vi "Wait For (str) (SubVI).vi"(1 "簇":T1={"initialize"=enum."SR830", "6221"={"6221 Resource"="GPIB0::24::INSTR", "Delta status"=FALSE, "电流"=0.0}, "SR830+6221"={"source"=0, "阻抗"=0.0, "量程入 4"=0, "量程入 3"=0, "量程入 2"=0, "量程入 1"=0, "SR830 2"=FALSE, "SR830 3"=FALSE, "SR830 4"=FALSE, "SR830 1"=FALSE, "VISA 1"="", "VISA 2"="", "VISA 3"="", "VISA 4"="", "Reserve 1"=0, "Reserve 2"=-1, "Reserve 3"=-1, "Reserve 4"=-1, "量程"=enum."量程每次测量会判定"}, "2400"={"2400"=FALSE, "VISA"=""}, "ch"={"ch"=[], "current"=[], "change?"=[], "holding current\nwhen change ch?"=FALSE}, "Instrument"={"335 Resource"="GPIB0::24::INSTR", "Input (0:A)"=0, "Instrument Type"=enum."SVSM", "quantum design"=refnum, "Heater Output (1:1)"=1, "semaphore"=refnum, "TCP master instance"=refnum, "335 Status"=refnum, "M24C Resource"="GPIB0::24::INSTR", "4G supply"="GPIB0::24::INSTR", "Temp Status 24C"=refnum, "4g supply status"=refnum, "Temp"=refnum}, "Aborting"=refnum, "数据文件"=refnum} {"Instrument"."Input (0:A)" items=["A", "B"]; "Instrument"."Heater Output (1:1)" items=["1"=1, "2"=2]; "SR830+6221"."Reserve 4" items=["Auto Reserve"=-1, "High Reserve"=0, "Normal"=1, "Low Noise"=2]; "SR830+6221"."Reserve 3" items=["Auto Reserve"=-1, "High Reserve"=0, "Normal"=1, "Low Noise"=2]; "SR830+6221"."Reserve 2" items=["Auto Reserve"=-1, "High Reserve"=0, "Normal"=1, "Low Noise"=2]; "SR830+6221"."Reserve 1" items=["量程每次测量会判定", "量程不变为设定值"]; "SR830+6221"."source" items=["SR830 1", "SR830 2", "SR830 3", "SR830 4"]}, 2 "字符串":string, 3 "error out":errorcluster) -> (10 "错误输出":errorcluster)   [LabVIEW 2019, in "Take Seq.lvlib"]
uses:
  Take Seq.lvlib
  <vilib>/NI/Modbus Library/API/Master/Modbus Master.lvclass
  config.ctl
  initialize.ctl
  Instrument.ctl
  Instrument Type.ctl
  lib/QDInstrument.dll
  335 state.ctl
  SubVI.lvlib
  9T cmag.lvlib
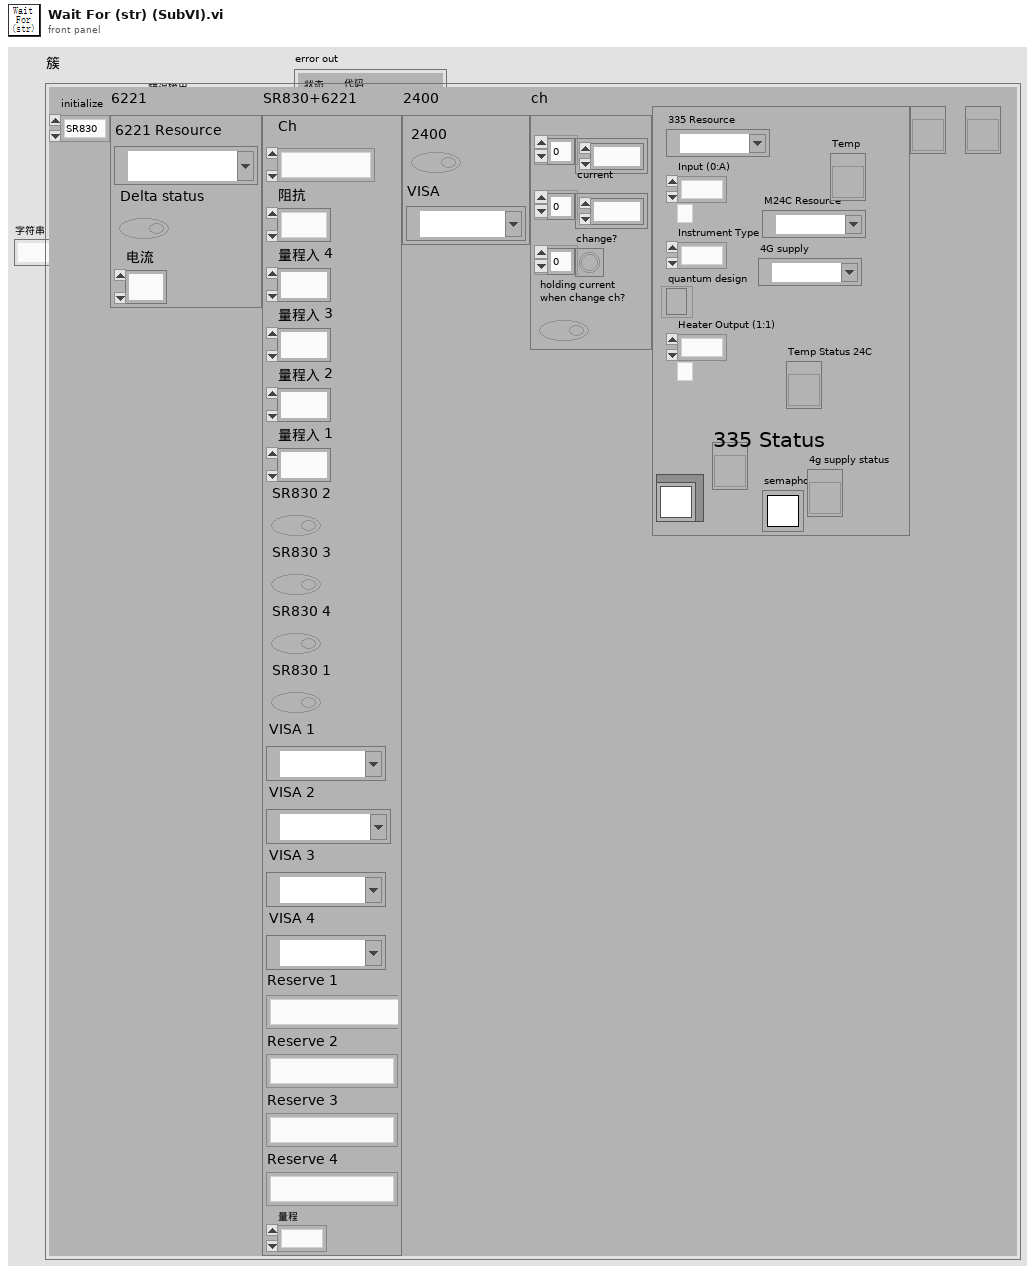
[diagram p1: front panel]
types:
  T1 = typedef "config.ctl" = cluster{"initialize":T2, "6221":cluster{"6221 Resource":refnum<visa-resource-name>, "Delta status":bool, "电流":dbl}, "SR830+6221":cluster{"source":u16, "阻抗":dbl, "量程入 4":i32, "量程入 3":i32, "量程入 2":i32, "量程入 1":i32, "SR830 2":bool, "SR830 3":bool, "SR830 4":bool, "SR830 1":bool, "VISA 1":refnum<visa-resource-name>, "VISA 2":refnum<visa-resource-name>, "VISA 3":refnum<visa-resource-name>, "VISA 4":refnum<visa-resource-name>, "Reserve 1":i16, "Reserve 2":i16, "Reserve 3":i16, "Reserve 4":i16, "量程":enum16{"量程每次测量会判定", "量程不变为设定值"}}, "2400":cluster{"2400":bool, "VISA":refnum<visa-resource-name>}, "ch":cluster{"ch":i32[], "current":dbl[], "change?":bool[], "holding current\nwhen change ch?":bool}, "Instrument":T3, "Aborting":refnum<vi>, "数据文件":refnum<vi>}
  T2 = typedef "initialize.ctl" = enum16{"SR830", "keithley6221-SR830", "Delta", "Delta-tunnelling", "keithley6221-2182-DC"}
  T3 = typedef "Instrument.ctl" = cluster{"335 Resource":refnum<visa-resource-name>, "Input (0:A)":u16, "Instrument Type":T4, "quantum design":refnum<k24>, "Heater Output (1:1)":u16, "semaphore":T5, "TCP master instance":refnum<class "Modbus Master.lvclass">, "335 Status":refnum<vi>, "M24C Resource":refnum<visa-resource-name>, "4G supply":refnum<visa-resource-name>, "Temp Status 24C":refnum<vi>, "4g supply status":refnum<vi>, "Temp":refnum<vi>}
  T4 = typedef "Instrument Type.ctl" = enum16{"PPMS", "VersaLab", "DynaCool", "SVSM", "PPMS-Rotate", "Lakeshore335", "9T mag"}
  T5 = typedef "Semaphore RefNum" = refnum<k1>
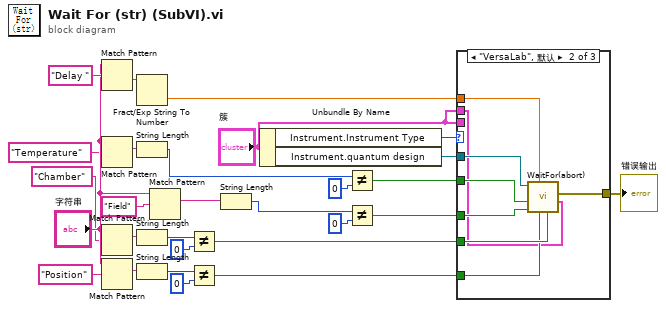
[diagram p0: block diagram]
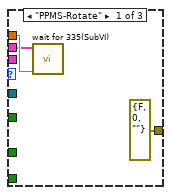
[diagram p2: hidden frame]
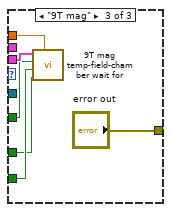
[diagram p3: hidden frame]
diagram:
  n1 = Match Pattern(string="字符串", regular expression="Delay " ("正则表达式")) -> (after substring=w24:string)  [unwired: 1 in, 3 out]
  n2 = Match Pattern(string="字符串", regular expression="Temperature" ("正则表达式")) -> (match substring=w4:string)  [unwired: 1 in, 3 out]
  n3 = Match Pattern(string="字符串", regular expression="Chamber" ("正则表达式")) -> (match substring=w14:string)  [unwired: 1 in, 3 out]
  n4 = Match Pattern(string="字符串", regular expression="Position" ("正则表达式")) -> (match substring=w11:string)  [unwired: 1 in, 3 out]
  n5 = Fract/Exp String To Number(string=w24) -> (number=w25:dbl)  [unwired: 3 in, 1 out]
  n6 = String Length(string=w4) -> (length=w5:i32)
  n7 = String Length(string=w14) -> (length=w15:i32)
  n8 = String Length(string=w11) -> (length=w12:i32)
  n9 = Match Pattern(string="字符串", regular expression="Field" ("正则表达式")) -> (match substring=w8:string)  [unwired: 1 in, 3 out]
  n10 = Not Equal?(x=w15, y=0) -> (x != y?=w27:bool)
  n11 = Not Equal?(x=w12, y=0) -> (x != y?=w26:bool)
  n12 = String Length(string=w8) -> (length=w9:i32)
  n13 = Unbundle By Name("簇") -> ("Instrument.Instrument Type"=w3:T4, "Instrument.quantum design"=w2:refnum<k24>)
  n14 = Not Equal?(x=w5, y=0) -> (x != y?=w7:bool)
  n15 = Not Equal?(x=w9, y=0) -> (x != y?=w21:bool)
  n16 = case shown="\"VersaLab\", 默认" w3 {
    tunnel: [errorcluster {"status"=FALSE, "code"=0, "source"=""} ("error out") w39 "error out"] -> w28
    tunnel: w27 -> [_ w38 w42]
    tunnel: w26 -> [_ w37 _]
    tunnel: w25 -> [w31 w36 w44]
    tunnel: w21 -> [_ w35 w41]
    tunnel: w7 -> [_ w34 w43]
    tunnel: w2 -> [_ w33 _]
    tunnel: "簇" -> [_ _ w45]
    tunnel: "簇" -> [w29 w32 _]
    frame "PPMS-Rotate" {
      n17 = call "wait for 335(SubVI).vi"("簇"=w29, "delay"=w31) -> ()  [unwired: 9 in]
    }
    frame "VersaLab", Default {
      n18 = call "WaitFor(abort).vi"("簇"=w32, "Wait For Chamber"=w38, "Wait For Position"=w37, "Delay"=w36, "Wait For Field"=w35, "Wait For Temperature"=w34, "Instrument Ref In"=w33) -> ("error out"=w39:errorcluster)  [unwired: 3 in, 1 out]
    }
    frame "9T mag" {
      n19 = call "9T mag temp-field-chamber wait for.vi"("delay"=w44, "Field"=w41, "Chamber"=w42, "temp"=w43, "输出簇"=w45) -> ()  [unwired: 7 in]
    }
  }
  "错误输出" <- w28
